vi "addChangeSTLs.vi"(8 "error in (no error)":errorcluster, 9 "Job Directory":path, 10 "STLs":cluster{"coordSys":T1, "WD":dbl, "STL":string}[](array[cluster]), 11 "parentObjectIn":refnum<vi>) -> (0 "error out":errorcluster, 3 "parentObjectOut":refnum<vi>, 4 "tunstlBits":refnum<vi>[](array[refnum]), 5 "TTstlBits":refnum<vi>[](array[refnum]), 6 "tunnelRef":refnum<vi>, 7 "turntableRef":refnum<vi>)   [LabVIEW 2022 SP3]
uses:
  coordSys.ctl
  ffa1697b-daa4-4c4c-a2b3-6e1e424d2b66.vi
  044be25f-ffbe-5747-992d-f4b49cc5da5d.vi
  <vilib>/picture/3D Picture Control/Object/Create Object (name).vi
  <vilib>/picture/3D Picture Control/Object/Add Object (reference).vi
  <vilib>/picture/3D Picture Control/NI_3D Picture Control.lvlib
panel:
  out "t":string
  out "Name":string
  out "notRefnum":bool
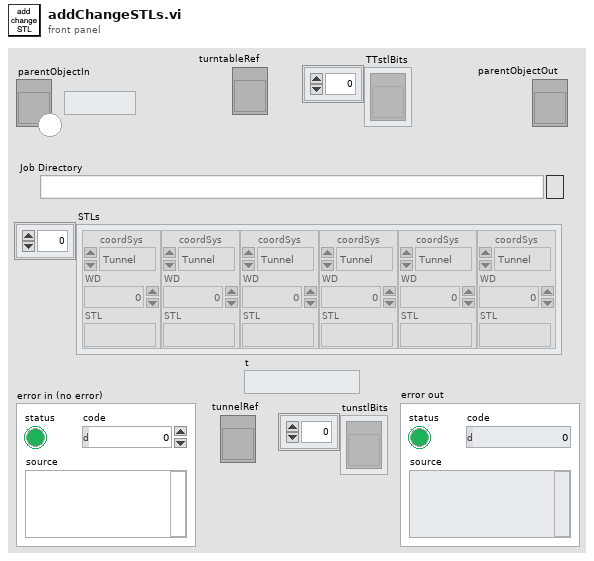
[diagram p1: front panel]
types:
  T1 = typedef "coordSys.ctl" = enum16{"Tunnel", "Model"}
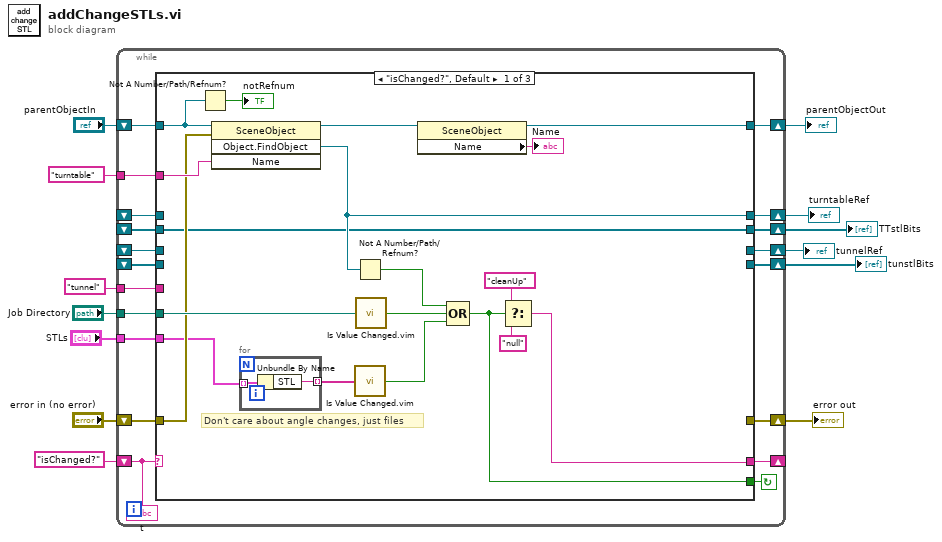
[diagram p0: block diagram]
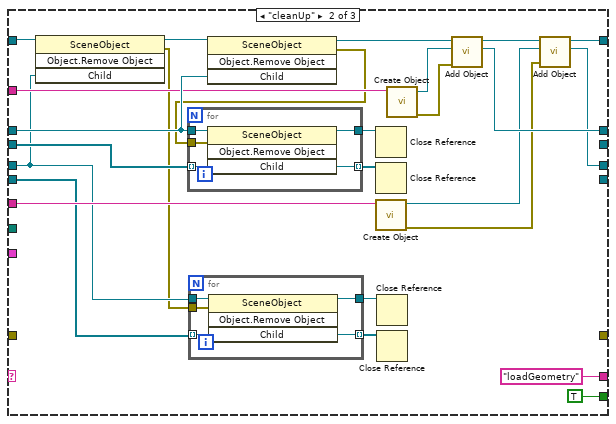
[diagram p2: hidden frame]
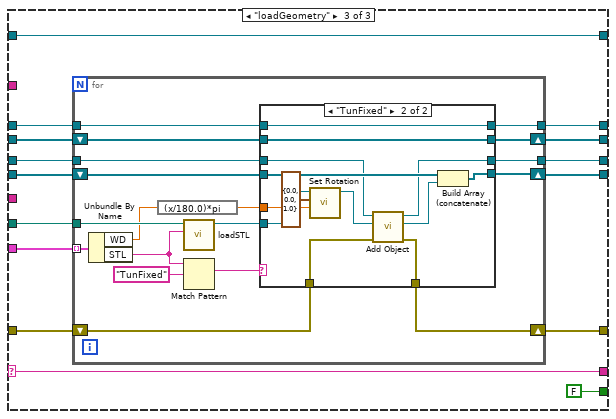
[diagram p3: hidden frame]
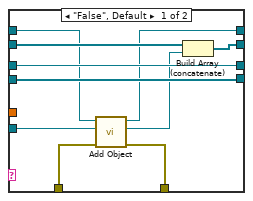
[diagram p4: hidden frame]
diagram:
  n1 = while {
    tunnel: "STLs" -> [w32]
    shift-right: [w24] -> _
    shift-left: "isChanged?" -> [w31]
    tunnel: "Job Directory" -> [w30]
    tunnel: "turntable" ("Name") -> [w28]
    shift-right: [w27] -> w10
    shift-left: _ -> [w26]
    shift-right: [w25] -> w9
    shift-left: "parentObjectIn" -> [w29]
    shift-right: [w21] -> w5
    shift-left: "error in (no error)" -> [w22]
    shift-right: [w20] -> w4
    shift-left: _ -> [w19]
    shift-right: [w15] -> w1
    shift-left: _ -> [w17]
    shift-right: [w18] -> w3
    shift-left: _ -> [w16]
    tunnel: "tunnel" ("Name") -> [w14]
    stop <- w23 continue-if-true
    n2 = case shown="\"isChanged?\", Default" w31 {
      selector: w31 -> [_ _ w98]
      tunnel: w32 -> [w34 _ w100]
      tunnel: w30 -> [w51 _ w101]
      tunnel: w29 -> [w39 w58 w95]
      tunnel: w28 -> [w47 w73 _]
      tunnel: [w44 w69 w94] -> w27
      tunnel: w26 -> [_ w76 w93]
      tunnel: [w36 w66 w95] -> w25
      tunnel: [w43 "loadGeometry" ("t") w98] -> w24
      tunnel: [w42 TRUE FALSE] -> w23
      tunnel: w22 -> [w41 _ w92]
      tunnel: [_ _ w97] -> w21
      tunnel: [w40 _ w96] -> w20
      tunnel: w19 -> [w40 w75 w90]
      tunnel: [_ _ w91] -> w18
      tunnel: w17 -> [_ w56 w89]
      tunnel: w16 -> [_ w60 w88]
      tunnel: [_ w63 w87] -> w15
      tunnel: w14 -> [_ w61 _]
      frame "isChanged?", Default {
        # "Don't care about angle changes, just files"
        n3 = Not A Number/Path/Refnum?(number/path/refnum=w39) -> (NaN/Path/Refnum?=→"notRefnum":bool)
        n4 = invoke class="SceneObject" method="Object.FindObject"(reference=w39, error in=w41, "Name"=w47) -> (reference out=w37:refnum<vi>, "FindObject"=w44:refnum<vi>)  [unwired: 1 in, 2 out]
        n5 = for {
          tunnel: w34 -> [w53] mode=indexing
          tunnel: [w52] -> w33 mode=indexing
          n6 = Unbundle By Name(w53) -> ("STL"=w52:string)
        }
        n7 = Not A Number/Path/Refnum?(number/path/refnum=w44) -> (NaN/Path/Refnum?=w46:bool)
        n8 = call "Is Value Changed.vim"("value"=w33) -> ("changed or first call?"=w49:bool)
        n9 = call "Is Value Changed.vim"("value"=w51) -> ("changed or first call?"=w50:bool)
        n10 = property class="SceneObject"(reference=w37) -> (reference out=w36:refnum<vi>, "Name"=→"Name":string)  [unwired: 1 in, 1 out]
        n11 = Compound Arithmetic op=OR(w46, w50, w49) -> (w42:bool)
        n12 = Select(t="cleanUp", s=w42, f="null") -> (s? t:f=w43:string)
      }
      frame "cleanUp" {
        n13 = invoke class="SceneObject" method="Object.Remove Object"(reference=w58, "Child"=w56) -> (reference out=w57:refnum<vi>, error out=w55:errorcluster)  [unwired: 2 in, 2 out]
        n14 = for {
          tunnel: w56 -> [w82]
          tunnel: w60 -> [w81] mode=indexing
          tunnel: [w81] -> w64 mode=indexing
          tunnel: [w80] -> w65
          tunnel: w55 -> [w79]
          n15 = invoke class="SceneObject" method="Object.Remove Object"(reference=w82, error in=w79, "Child"=w81) -> (reference out=w80:refnum<vi>)  [unwired: 1 in, 3 out]
        }
        n16 = invoke class="SceneObject" method="Object.Remove Object"(reference=w57, "Child"=w76) -> (reference out=w72:refnum<vi>, error out=w54:errorcluster)  [unwired: 2 in, 2 out]
        n17 = for {
          tunnel: w76 -> [w86]
          tunnel: w75 -> [w85] mode=indexing
          tunnel: [w85] -> w74 mode=indexing
          tunnel: [w84] -> w68
          tunnel: w54 -> [w83]
          n18 = invoke class="SceneObject" method="Object.Remove Object"(reference=w86, error in=w83, "Child"=w85) -> (reference out=w84:refnum<vi>)  [unwired: 1 in, 3 out]
        }
        n19 = Close Reference(reference=w68) -> ()  [unwired: 1 in, 1 out]
        n20 = Close Reference(reference=w74) -> ()  [unwired: 1 in, 1 out]
        n21 = call-poly <vilib>:"Create Object.vi"("Name"=w61) -> ("error out"=w59:errorcluster, "Scene:New Object"=w62:refnum<vi>)  [unwired: 9 in]
        n22 = Close Reference(reference=w65) -> ()  [unwired: 1 in, 1 out]
        n23 = Close Reference(reference=w64) -> ()  [unwired: 1 in, 1 out]
        n24 = call-poly <vilib>:"Create Object.vi"("Name"=w73) -> ("error out"=w70:errorcluster, "Scene:New Object"=w71:refnum<vi>)  [unwired: 9 in]
        n25 = call-poly <vilib>:"Add Object.vi"("error in (no error)"=w70, "New Object In"=w71, "Scene Object In"=w72) -> ("New Object Out"=w69:refnum<vi>, "Scene Object Out"=w67:refnum<vi>)  [unwired: 6 in, 1 out]
        n26 = call-poly <vilib>:"Add Object.vi"("error in (no error)"=w59, "New Object In"=w62, "Scene Object In"=w67) -> ("New Object Out"=w63:refnum<vi>, "Scene Object Out"=w66:refnum<vi>)  [unwired: 6 in, 1 out]
      }
      frame "loadGeometry" {
        n27 = for {
          tunnel: w101 -> [w118]
          tunnel: w100 -> [w119] mode=indexing
          shift-right: [w104] -> w97
          shift-left: w92 -> [w106]
          shift-right: [w110] -> w91
          shift-left: w88 -> [w108]
          shift-right: [w112] -> w96
          shift-left: w90 -> [w111]
          tunnel: w93 -> [w114]
          tunnel: [w113] -> w94
          tunnel: w89 -> [w109]
          tunnel: [w107] -> w87
          n28 = Unbundle By Name(w119) -> ("WD"=w102:dbl, "STL"=w116:string)
          n29 = expression code="(x/180.0)*pi" ("degrees to radians")(w102) -> (w103:dbl)
          n30 = call "loadSTL.vi"("STLname"=w116, "Job Directory"=w118) -> ("SceneObject out"=w105:refnum<vi>)  [unwired: 8 in, 1 out]
          n31 = Match Pattern(string=w116, regular expression="TunFixed") -> (match substring=w115:string)  [unwired: 1 in, 3 out]
          n32 = case shown="\"TunFixed\"" w115 {
            tunnel: w114 -> [w121 w140]
            tunnel: [w122 w140] -> w113
            tunnel: [w129 w142] -> w112
            tunnel: w111 -> [w128 w142]
            tunnel: [w126 w141] -> w110
            tunnel: w109 -> [w127 w134]
            tunnel: w108 -> [w126 w139]
            tunnel: [w127 w135] -> w107
            tunnel: w106 -> [w124 w138]
            tunnel: w105 -> [w125 w132]
            tunnel: [w123 w137] -> w104
            tunnel: w103 -> [_ w130]
            frame "False", Default {
              n33 = call-poly <vilib>:"Add Object.vi"("error in (no error)"=w124, "New Object In"=w125, "Scene Object In"=w121) -> ("error out"=w123:errorcluster, "New Object Out"=w120:refnum<vi>, "Scene Object Out"=w122:refnum<vi>)  [unwired: 6 in]
              n34 = Build Array (concatenate)(w128, w120) -> (w129:refnum<vi>[])
            }
            frame "TunFixed" {
              n35 = call <vilib>:"Set Rotation.vi"("Angle"=w130, "Axis"=cluster{"X":sgl, "Y":sgl, "Z":sgl} {"X"=0.0, "Y"=0.0, "Z"=1.0}, "Scene Object"=w132) -> ("Rotated Scene Object"=w133:refnum<vi>)  [unwired: 7 in, 1 out]
              n36 = call-poly <vilib>:"Add Object.vi"("error in (no error)"=w138, "New Object In"=w133, "Scene Object In"=w134) -> ("error out"=w137:errorcluster, "New Object Out"=w136:refnum<vi>, "Scene Object Out"=w135:refnum<vi>)  [unwired: 6 in]
              n37 = Build Array (concatenate)(w139, w136) -> (w141:refnum<vi>[])
            }
          }
        }
      }
    }
    "t" <- w31
  }
  "turntableRef" <- w10
  "parentObjectOut" <- w9
  "error out" <- w5
  "TTstlBits" <- w4
  "tunstlBits" <- w3
  "tunnelRef" <- w1
